vi "Params string to array.vi"(10 "String params":string) -> (0 "Last":string, 2 "Array of params":string[](array[string]))   [LabVIEW 2021, in "STAV lib.lvlib"]
uses:
  STAV lib.lvlib
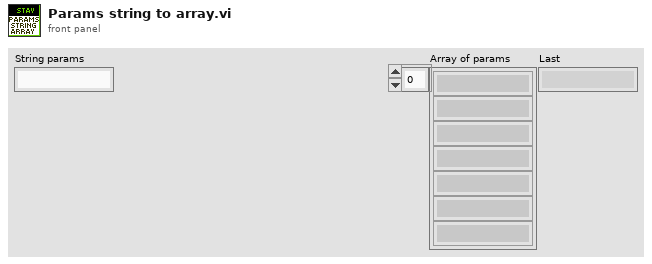
[diagram p1: front panel]
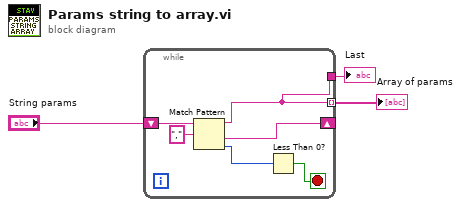
[diagram p0: block diagram]
diagram:
  n1 = while {
    shift-right: [w8] -> _
    shift-left: "String params" -> [w9]
    tunnel: [w4] -> w2 mode=indexing
    tunnel: [w4] -> w1
    stop <- w7 stop-if-true
    n2 = Match Pattern(string=w9, regular expression=",") -> (before substring=w4:string, after substring=w8:string, offset past match=w6:i32)  [unwired: 1 in, 1 out]
    n3 = Less Than 0?(x=w6) -> (x < 0?=w7:bool)
  }
  "Array of params" <- w2
  "Last" <- w1
